vi "Status DL.vi"(8 "error in (no error)":errorcluster, 10 "data":variant, 11 "Control-Client in":refnum<class "Control-Client.lvclass">) -> (0 "error out":errorcluster, 2 "error IO":errorcluster, 3 "Control-Client out":refnum<class "Control-Client.lvclass">)   [LabVIEW 2019, in "Control-Client.lvclass"]
uses:
  Control-Client.lvclass
  dependecies/ControlsVIs/Clusters-def/Commands-CLIENT.ctl
  dependecies/ControlsVIs/Clusters-def/Message types.ctl
  dependecies/ControlsVIs/Clusters-def/DL-Reply-to-Connect-to-Client.ctl
  Delay Line/DelayLine.lvclass
  Message/Message.lvclass
  dependecies/XControls/CellsDL/ControlDL.xctl
  GeneralFunctionality/GeneralFunctionality.lvclass
  C:/dev/TRANCON/Classes/GeneralFunctionality/GeneralFunctionality.lvclass
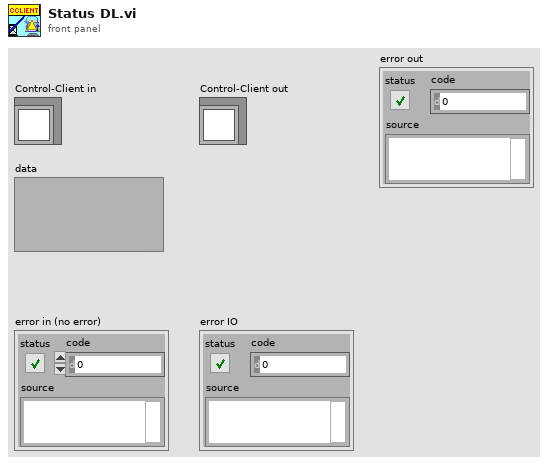
[diagram p1: front panel]
types:
  T1 = typedef "DelayLine.lvclass/DL-Reply-to-Connect-to-Client.ctl" = cluster{"on/off":bool, "pos":dbl[], "param":cluster{"min":dbl, "max":dbl, "real pos":dbl}[], "predefine_pos":dbl[][], "error":errorcluster}
  T2 = typedef "Message types.ctl" = string
  T3 = typedef "Control-Client.lvclass/Commands-CLIENT.ctl" = string
  T4 = cluster{"min I, mm":dbl, "max I, mm":dbl, "Optical 0, ps":dbl, "min II, mm":dbl, "max II, mm ":dbl}
  T5 = typedef "Control-Client.lvclass/Controls-with-permissions_CLIENT.ctl" = cluster{"Server ON/OFF":refnum<vi>, "Detector connect":refnum<vi>, "DL connect":refnum<vi>, "DAQmx connect":refnum<vi>, "All connect":refnum<vi>, "Start measurement":refnum<vi>, "Move Crystal":refnum<vi>, "Relay key heater":refnum<vi>, "Laser Shutter":refnum<vi>, "Accelerator Shutter":refnum<vi>, "Power":refnum<vi>, "Unlock":refnum<vi>, "RT":refnum<vi>, "Faraday Cup":refnum<vi>, "Osc connect":refnum<vi>, "ELYSE pulses":refnum<vi>, "Cells":refnum<vi>, "Pump":refnum<vi>, "# par point":refnum<vi>, "Alarm":refnum<vi>, "oscilloscopeRead":refnum<vi>, "WCM_state":refnum<vi>, "ControlDL":refnum<vi>}
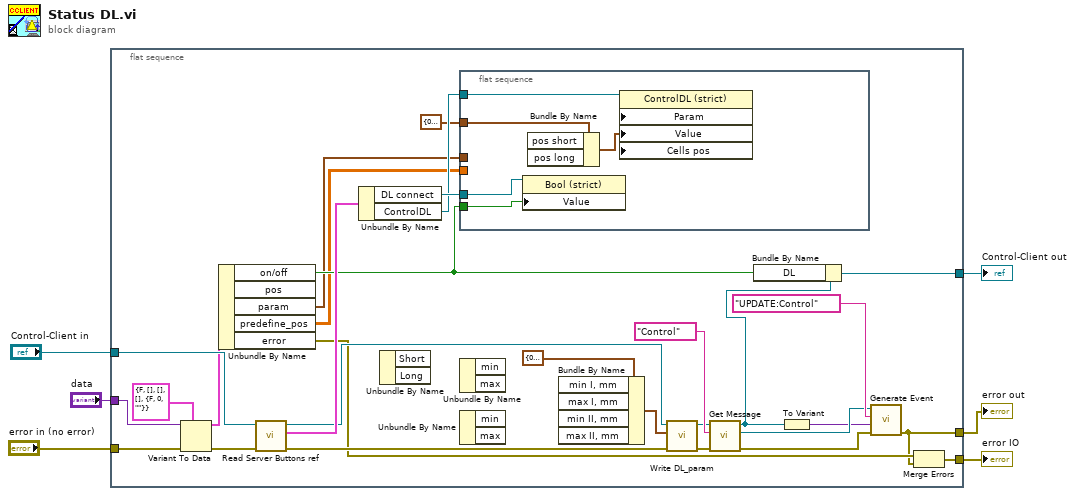
[diagram p0: block diagram]
diagram:
  n1 = flat-sequence {
    tunnel: "data" -> [w35]
    tunnel: "Control-Client in" -> [w34]
    tunnel: "error in (no error)" -> [w32]
    tunnel: [w12] -> w5
    tunnel: [w14] -> w6
    tunnel: [w10] -> w1
    frame #0 {
      n2 = Variant To Data(error in=w32, type=T1 {"on/off"=FALSE, "pos"=[], "param"=[], "predefine_pos"=[], "error"={"status"=FALSE, "code"=0, "source"=""}} ("output cluster"), Variant=w35) -> (data=w29:T1, error out=w33:errorcluster)
      n3 = Unbundle By Name(w29) -> ("on/off"=w11:bool, "param"=w8:cluster{"min":dbl, "max":dbl, "real pos":dbl}[], "predefine_pos"=w7:dbl[][], "error"=w15:errorcluster)  [unwired: 1 out]
      n4 = call "Read Server Buttons ref.vi"("error in (no error)"=w33, "Control-Client in"=w34) -> ("error out"=w26:errorcluster, "Server Buttons ref"=w31:T5, "Control-Client out"=w27:refnum<class "Control-Client.lvclass">)  [unwired: 7 in]
      n5 = Unbundle By Name(w31) -> ("DL connect"=w30:refnum<vi>, "ControlDL"=w16:refnum<vi>)
      n6 = Unbundle By Name() -> ()  [unwired: 1 in, 2 out]
      n7 = flat-sequence {
        tunnel: w30 -> [w40]
        tunnel: w16 -> [w39]
        tunnel: w11 -> [w38]
        tunnel: cluster{"pos short":dbl, "pos long":dbl} {"pos short"=0.0, "pos long"=0.0} ("Valeur") -> [w37]
        tunnel: w8 -> [_]
        tunnel: w7 -> [_]
        frame #0 {
          n8 = property class="Bool (strict)"(reference=w40, "Value"=w38) -> ()  [unwired: 1 in, 2 out]
          n9 = Bundle By Name(cluster=w37) -> (w36:cluster{"pos short":dbl, "pos long":dbl})  [unwired: 2 in]
          n10 = property class="ControlDL (strict)" props=["Param", "Value", "Cells pos"](reference=w39, "Value"=w36) -> ()  [unwired: 3 in, 2 out]
        }
      }
      n11 = Unbundle By Name() -> ()  [unwired: 1 in, 2 out]
      n12 = Unbundle By Name() -> ()  [unwired: 1 in, 2 out]
      n13 = Bundle By Name(cluster=T4 {"min I, mm"=0.0, "max I, mm"=0.0, "Optical 0, ps"=0.0, "min II, mm"=0.0, "max II, mm "=0.0} ("DL_param")) -> (w24:T4)  [unwired: 4 in]
      n14 = call "Write DL_param.vi"("error in (no error)"=w26, "DL_param"=w24, "Control-Client in"=w27) -> ("error out"=w19:errorcluster, "Control-Client out"=w17:refnum<class "Control-Client.lvclass">)  [unwired: 7 in]
      n15 = call "Get Message.vi"("error in (no error)"=w19, "Message type"=T2 "Control", "GeneralFunctionality en entrée"=w17) -> ("error out"=w20:errorcluster, "Message.lvclass"=w22:refnum<class "Message.lvclass">, "GeneralFunctionality en sortie"=w13:refnum<class "Control-Client.lvclass">)  [unwired: 6 in]
      n16 = Bundle By Name(cluster=w13, "DL"=w11) -> (w12:refnum<class "Control-Client.lvclass">)
      n17 = To Variant(anything=w13) -> (Variant=w18:variant)
      n18 = call "Generate Event.vi"("error in (no error)"=w20, "Data"=w18, "Command"=T3 "UPDATE:Control" ("Commands-Client"), "Message en entrée"=w22) -> ("error out"=w10:errorcluster)  [unwired: 6 in, 1 out]
      n19 = Merge Errors(w15, w10) -> (w14:errorcluster)
    }
  }
  "error IO" <- w6
  "Control-Client out" <- w5
  "error out" <- w1
